vi "Main.vi"() -> ()   [LabVIEW 2010]
uses:
  <vilib>/Utility/miscctls.llb/LVMenuShortCut.ctl
  sub VIs v Hauptprogramm/globale Variable 1.vi
panel:
  out "version":string="1.5.1.1"
  in  "Stopp 2":bool
  in  "endgültigeschließung":bool
  in  "fehlbearbeitungen":i32
  out "Farbwerte":T1
  in  "farbe":bool
  out "stop2":bool
  out "hitze":u64(knob)=398 caption="lichtquellen Temparatur" scale=420.0..356.0
  in  "Not-Aus betätigt":dbl
  in  "bearbeitung gestartedt":dbl
  out "start zeit":timestamp
  in  "protokoll":bool
  out "Lampe Notaus":bool
  out "error out":errorcluster
  in  "pneutest":bool
  out "error out senke":errorcluster
  out "gesperrt?":bool
  in  "schließen":bool
  out "export?":bool
  in  "error in (no error)":errorcluster caption="Fehler (Eingang, kein Fehler)"
  in  "Licht":bool
  in  "Ende":bool
  out "Device ID Out":T2(ring)
  in  "Interfacetest":bool
  in  "Stopp":bool
  out "Zeitstempel":timestamp=timestamp(-9593251200 s since 1904-01-01) format="%<%H:%M:%S\n%d/%m/%Y>T"
  in  "Sperren":bool
  # "456"
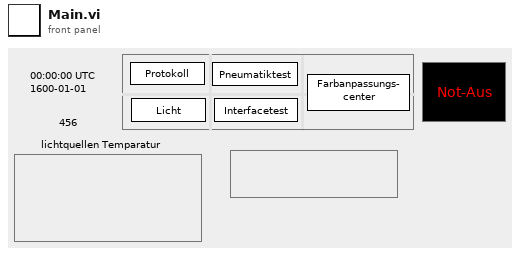
[diagram p1: front panel]
types:
  T1 = cluster{"Rot-min.":dbl, "Rot.max.":dbl, "Blau-min.":dbl, "Blau-max.":dbl, "Grün-min.":dbl, "Grün-max.":dbl, "Weiß-min.":dbl, "Weiß-max.":dbl}
  T2 = enum16{"Device 1", "Device 2", "Device 3", "Device 4", "Device 5", "Device 6", "Device 7", "Device 8"}
  T3 = enum8{"Power 1", "Power 2", "Power 3", "Power 4", "Power 5", "Power 6", "Power 7", "Power 8"}
  T4 = enum8{"Output 1 (O1)", "Output 2 (O2)", "Output 3 (O3)", "Output 4 (O4)", "Output 5 (O5)", "Output 6 (O6)", "Output 7 (O7)", "Output 8 (O8)"}
  T5 = enum8{"Robo Interface", "Extension 1", "Extension 2", "Extension 3"}
  T6 = enum8{"Input 1 (I1)", "Input 2 (I2)", "Input 3 (I3)", "Input 4 (I4)", "Input 5 (I5)", "Input 6 (I6)", "Input 7 (I7)", "Input 8 (I8)"}
  T7 = enum8{"Input AX", "Input AY", "Input A1", "Input A2", "Input AZ", "Input AV", "Input D1", "Input D2", "Input AXR", "Input AYR"}
  T8 = enum8{"Goes High", "Goes Low", "Goes High or Low"}
  T9 = typedef "LVMenuShortCut.ctl" = cluster{"Include Shift Key?":bool, "Include Ctrl Key?":bool, "Shortcut Key":string}
  T10 = enum8{"Robo Interface", "Extension 1", "Extension 2", "Extension 3"}[]
  T11 = enum8{"Input 1 (I1)", "Input 2 (I2)", "Input 3 (I3)", "Input 4 (I4)", "Input 5 (I5)", "Input 6 (I6)", "Input 7 (I7)", "Input 8 (I8)"}[]
  T12 = cluster{"Value[0]":bool, "Value[1]":bool, "Value[2]":bool, "Value[3]":bool, "Value[4]":bool, "Value[5]":bool, "Value[6]":bool, "Value[7]":bool, "Value[8]":bool}
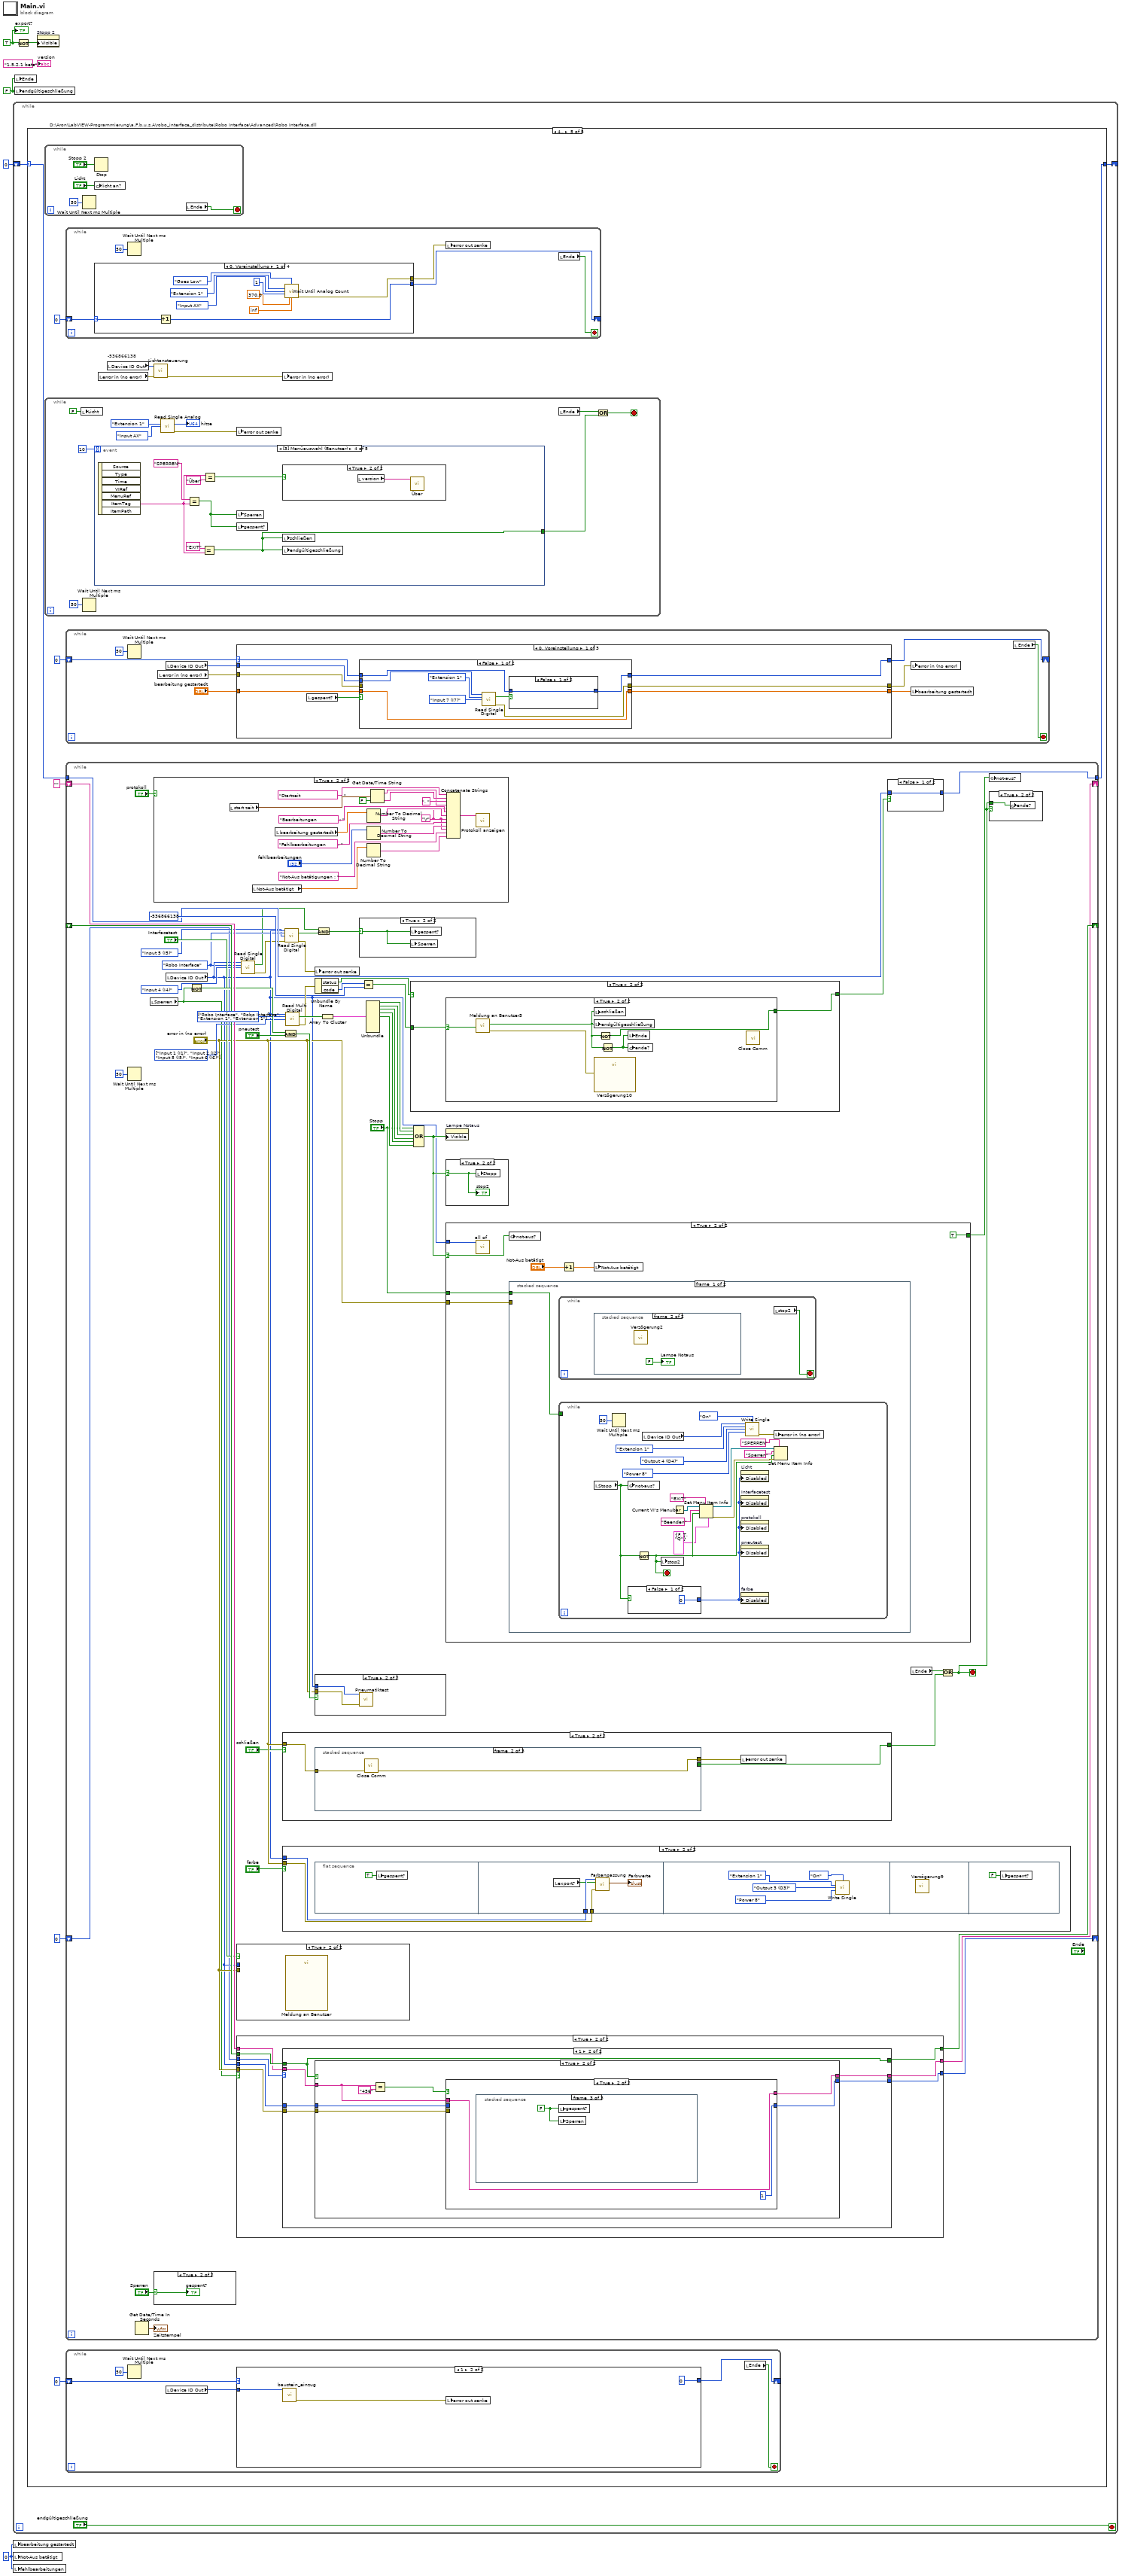
[diagram p0: block diagram]
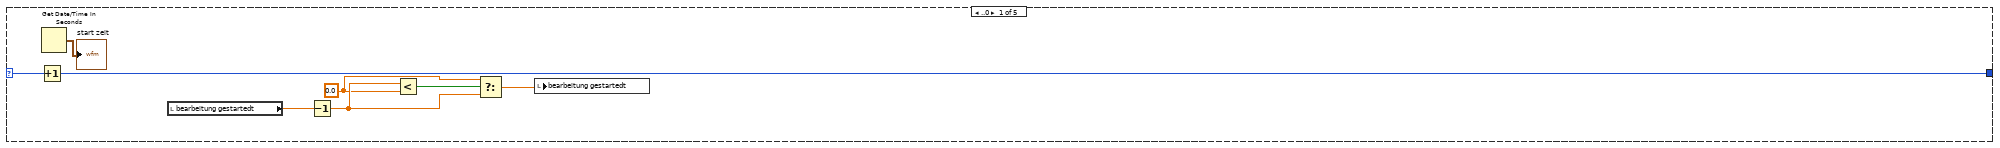
[diagram p2: hidden frame]
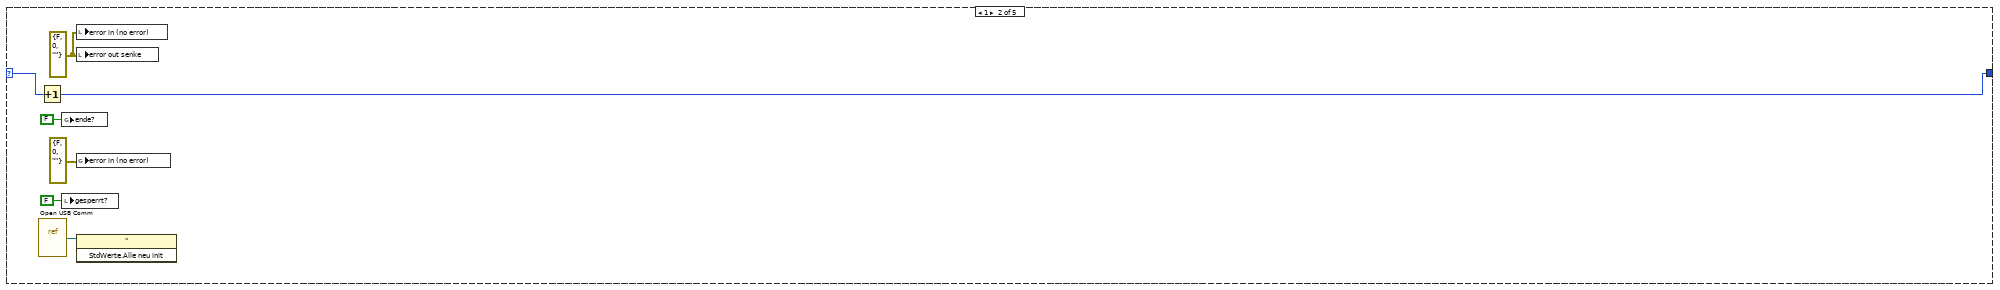
[diagram p3: hidden frame]
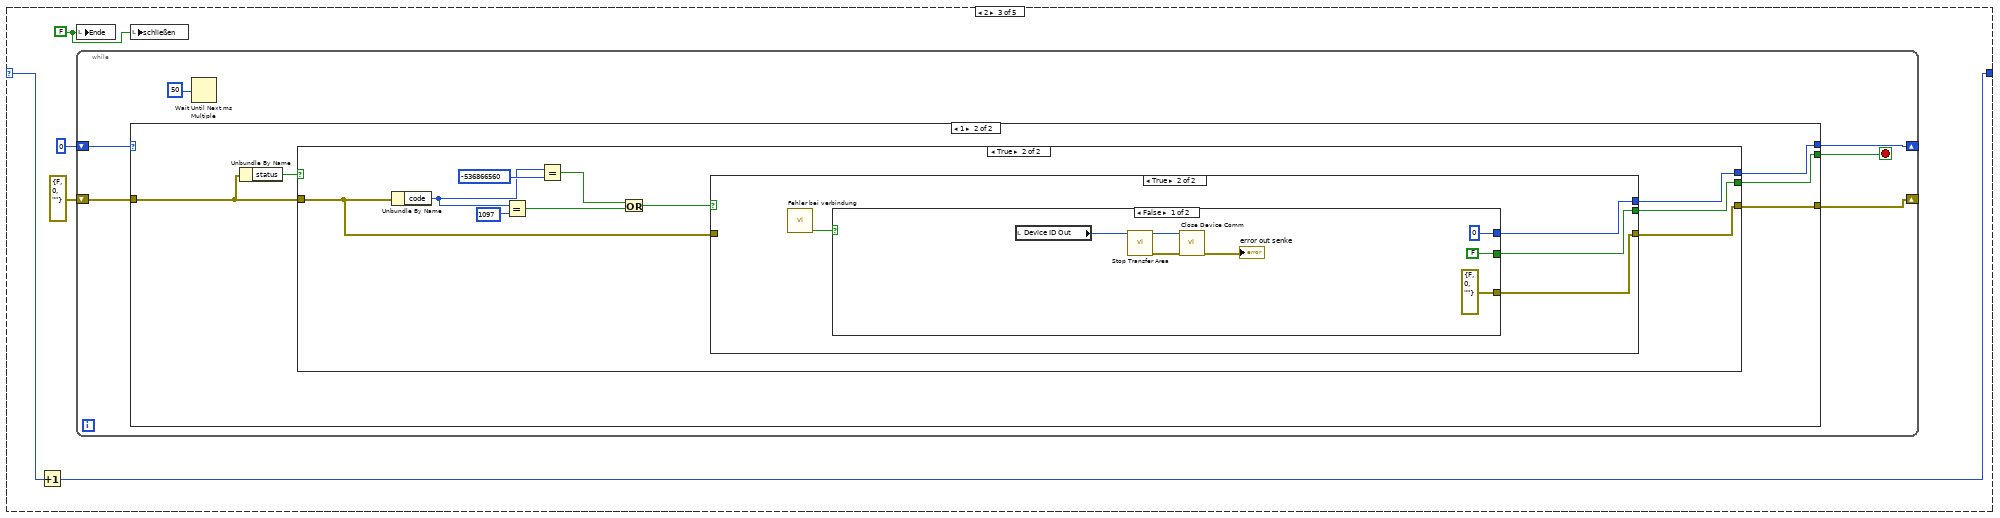
[diagram p4: hidden frame]
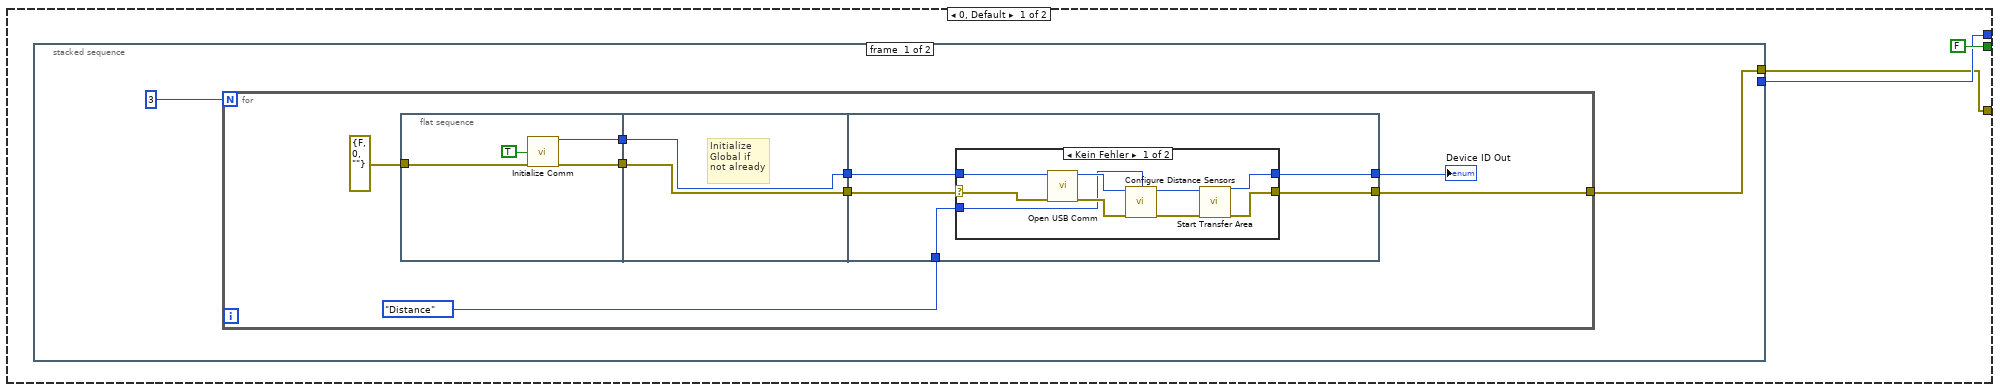
[diagram p5: hidden frame]
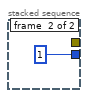
[diagram p7: hidden frame]
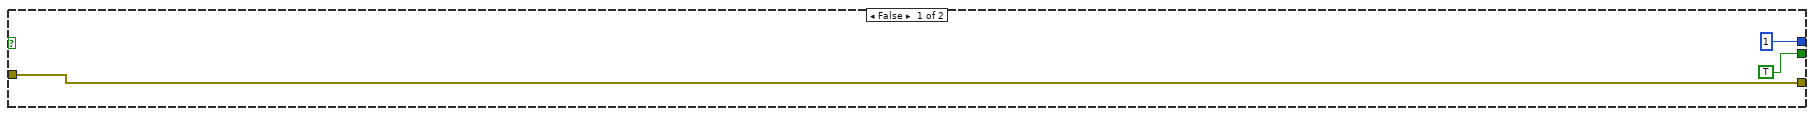
[diagram p8: hidden frame]
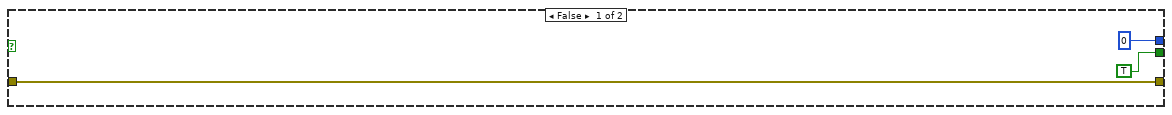
[diagram p9: hidden frame]
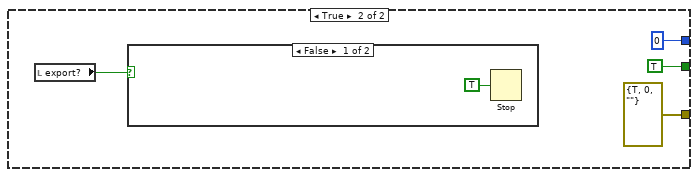
[diagram p10: hidden frame]
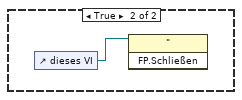
[diagram p11: hidden frame]
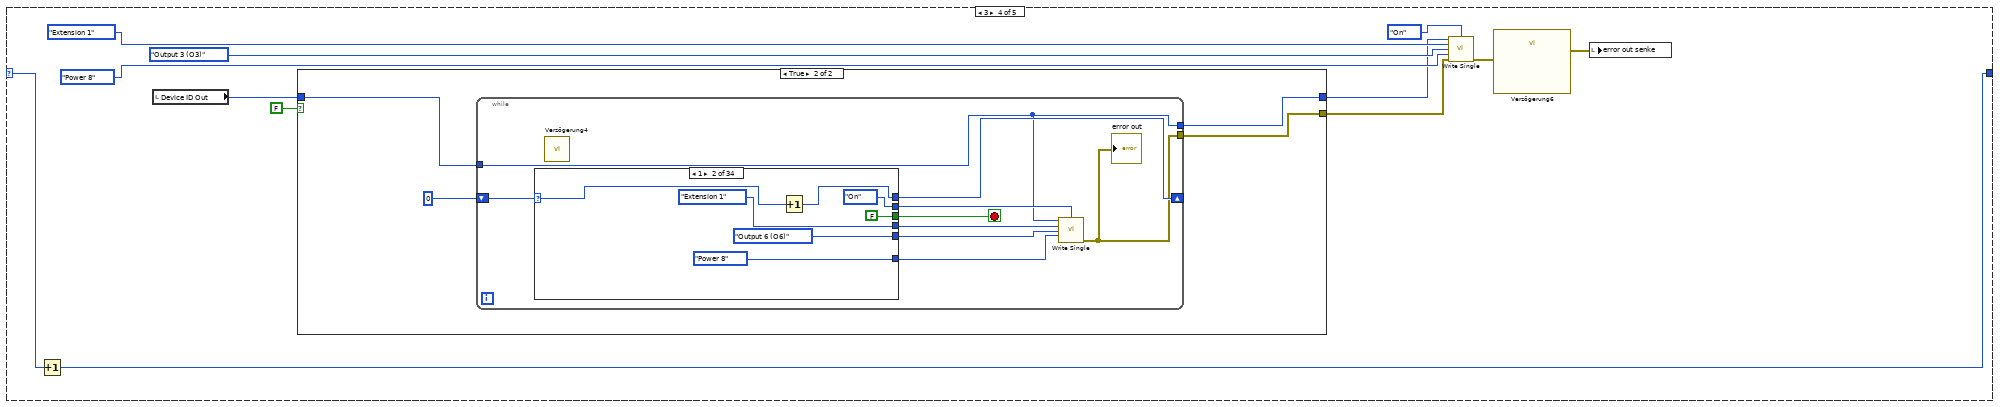
[diagram p12: hidden frame]
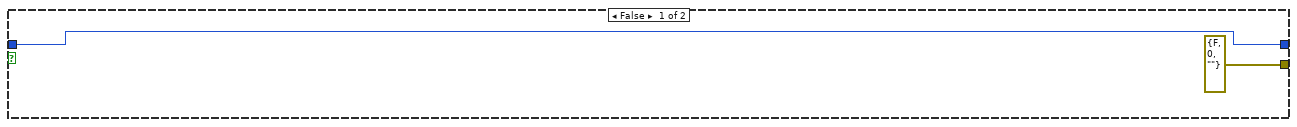
[diagram p13: hidden frame]
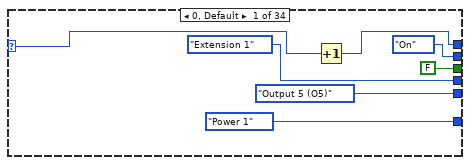
[diagram p14: hidden frame]
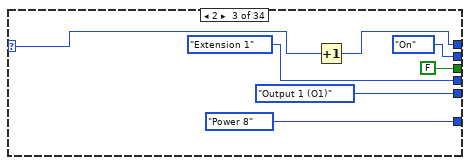
[diagram p15: hidden frame]
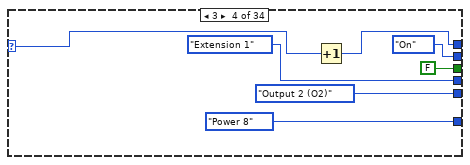
[diagram p16: hidden frame]
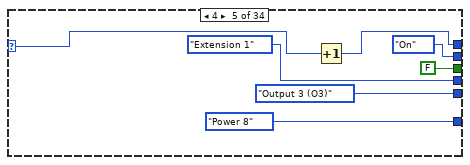
[diagram p17: hidden frame]
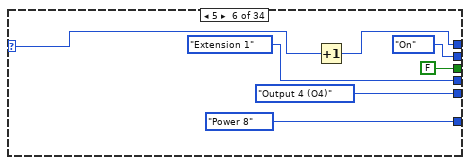
[diagram p18: hidden frame]
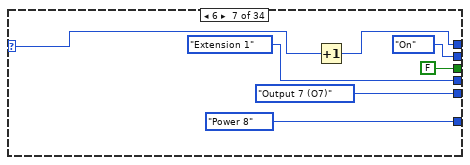
[diagram p19: hidden frame]
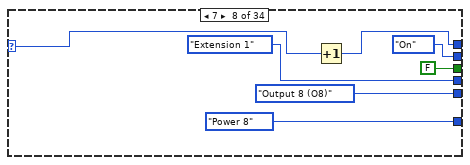
[diagram p20: hidden frame]
diagram:
  w4 = 0
  w5 = FALSE ("Ende")
  w3 = TRUE ("export?")
  n1 = while {
    shift-right: [w7] -> _
    shift-left: 0 -> [w9]
    stop <- "endgültigeschließung" stop-if-true
    # "D:\\Aron\\LabVIEW-Programmierung\\a.F.b.u.s.A\\robo_interface_distribute\\Robo Interface\\Advanced\\Robo Interface.dll"
    n2 = case shown="4.." w9 {
      selector: w9 -> [w16 w20 w25 w112 w376]
      tunnel: [w15 w19 w26 w111 w375] -> w7
      frame ..0 {
        w11 = 0.0 ("y")
        n3 = Increment(x=w16) -> (x+1=w15:i32)
        n4 = Get Date/Time In Seconds() -> (seconds since 1Jan1904=→"start zeit":timestamp)
        n5 = local read "bearbeitung gestartedt"() -> (w14:dbl)
        n6 = Decrement(x=w14) -> (x-1=w12:dbl)
        n7 = Less?(x=w12, y=w11) -> (x < y?=w13:bool)
        n8 = Select(t=w11, s=w13, f=w12) -> (s? t:f=w10:dbl)
        n9 = local write "bearbeitung gestartedt"(w10) -> ()
      }
      frame 1 {
        w21 = errorcluster {"status"=FALSE, "code"=0, "source"=""} ("error in (no error)")
        n10 = vi-ref "Open USB Comm.vi"() -> (w24:refnum<vi>)
        n11 = Increment(x=w20) -> (x+1=w19:i32)
        n12 = global write "globale Variable 1.vi" "ende?"(FALSE ("ende?")) -> ()
        n13 = local write "gesperrt?"(FALSE ("gesperrt?")) -> ()
        n14 = local write "error in (no error)"(w21) -> ()
        n15 = local write "error out senke"(w21) -> ()
        n16 = global write "globale Variable 1.vi" "error in (no error)"(errorcluster {"status"=FALSE, "code"=0, "source"=""} ("error in (no error)")) -> ()
        n17 = invoke class="\"" method="StdWerte.Alle neu init"(reference=w24) -> ()  [unwired: 2 in, 3 out]
      }
      frame 2 {
        w27 = FALSE
        n18 = Increment(x=w25) -> (x+1=w26:i32)
        n19 = local write "Ende"(w27) -> ()
        n20 = while {
          shift-right: [w32] -> _
          shift-left: 0 -> [w35]
          shift-right: [w34] -> _
          shift-left: errorcluster {"status"=FALSE, "code"=0, "source"=""} ("error out") -> [w33]
          stop <- w31 stop-if-true
          n21 = case shown="1" w35 {
            tunnel: [w36 w72] -> w34
            tunnel: w33 -> [_ w73]
            tunnel: [w37 w76] -> w32
            tunnel: [FALSE w74] -> w31
            frame 0, Default {
              n22 = stacked-sequence {
                tunnel: [_ 1] -> w37
                tunnel: [w40 _] -> w36
                frame #0 {
                  n23 = for {
                    N: 3 -> [_]
                    tunnel: [w41] -> w40
                    n24 = flat-sequence {
                      tunnel: [w52] -> w48
                      tunnel: [w51] -> w47
                      tunnel: errorcluster {"status"=FALSE, "code"=0, "source"=""} ("error in") -> [w50]
                      tunnel: [w54] -> w46
                      tunnel: [w53] -> w45
                      tunnel: w48 -> [w54]
                      tunnel: w47 -> [w53]
                      tunnel: w46 -> [w59]
                      tunnel: w45 -> [w58]
                      tunnel: [w57] -> w41
                      tunnel: [w56] -> w44
                      tunnel: enum32{"Voltage", "Distance"}."Distance" ("Distance Sensor Mode") -> [w55]
                      frame #0 {
                        n25 = call "Initialize Comm.vi"("immer erster aufruf?"=TRUE, "error in"=w50) -> ("Device ID Out"=w52:T2, "error out"=w51:errorcluster)  [unwired: 1 in, 11 out]
                      }
                      frame #1 {
                        # "Initialize\nGlobal if\nnot already"
                      }
                      frame #2 {
                        n26 = case shown="Kein Fehler" w58 {
                          selector: w58 -> [w65 w70]
                          tunnel: [w68 w70] -> w57
                          tunnel: w59 -> [w63 w69]
                          tunnel: [w67 w69] -> w56
                          tunnel: w55 -> [w61 _]
                          frame No Error {
                            n27 = call "Open USB Comm.vi"("Device ID"=w63, "error in"=w65) -> ("Device ID Out"=w62:T2, "error out"=w64:errorcluster)  [unwired: 12 out]
                            n28 = call "Configure Distance Sensors.vi"("Device ID"=w62, "Distance Sensor Mode"=w61, "error in"=w64) -> ("Device ID Out"=w60:T2, "error out"=w66:errorcluster)  [unwired: 6 in, 5 out]
                            n29 = call "Start Transfer Area.vi"("Device ID"=w60, "error in"=w66) -> ("Device ID Out"=w67:T2, "error out"=w68:errorcluster)  [unwired: 12 out]
                          }
                          frame Error {
                          }
                        }
                      }
                    }
                    "Device ID Out" <- w44
                  }
                }
                frame #1 {
                }
              }
            }
            frame 1 {
              n30 = Unbundle By Name(w73) -> ("status"=w75:bool)
              n31 = case shown="True" w75 {
                tunnel: w73 -> [w77 w88]
                tunnel: [1 w87] -> w76
                tunnel: [TRUE w86] -> w74
                tunnel: [w77 w85] -> w72
                frame False {
                }
                frame True {
                  n32 = Unbundle By Name(w88) -> ("code"=w84:i32)
                  n33 = Equal?(x=w84, y=1097) -> (x = y?=w82:bool)
                  n34 = Equal?(x=w84, y=-536866560) -> (x = y?=w83:bool)
                  n35 = Or(x=w83, y=w82) -> (x .or. y?=w81:bool)
                  n36 = case shown="True" w81 {
                    tunnel: w88 -> [w90 _]
                    tunnel: [0 w96] -> w87
                    tunnel: [TRUE w95] -> w86
                    tunnel: [w90 w94] -> w85
                    frame False {
                    }
                    frame True {
                      n37 = call "Fehler bei verbindung.vi"() -> ("schließen?"=w93:bool)  [unwired: 11 out]
                      n38 = case shown="False" w93 {
                        tunnel: [0 0] -> w96
                        tunnel: [FALSE TRUE] -> w95
                        tunnel: [errorcluster {"status"=FALSE, "code"=0, "source"=""} ("error out") errorcluster {"status"=TRUE, "code"=0, "source"=""} ("error out")] -> w94
                        frame False {
                          n39 = local read "Device ID Out"() -> (w99:T2)
                          n40 = call "Stop Transfer Area.vi"("Device ID"=w99) -> ("Device ID Out"=w100:T2, "error out"=w97:errorcluster)  [unwired: 1 in, 12 out]
                          n41 = call "Close Device Comm.vi"("Device ID"=w100, "error in"=w97) -> ("error out"=→"error out senke":errorcluster)  [unwired: 13 out]
                        }
                        frame True {
                          n42 = local read "export?"() -> (w104:bool)
                          n43 = case shown="False" w104 {
                            frame False {
                              n44 = Stop(stop? (T)=TRUE ("Stopp? (T)")) -> ()
                            }
                            frame True {
                              n45 = control-ref of="dieses VI"() -> (w109:refnum<vi>)
                              n46 = invoke class="\"" method="FP.Schließen"(reference=w109) -> ()  [unwired: 2 in, 3 out]
                            }
                          }
                        }
                      }
                    }
                  }
                }
              }
            }
          }
          n47 = Wait Until Next ms Multiple(millisecond multiple=50) -> ()  [unwired: 1 out]
        }
        n48 = local write "schließen"(w27) -> ()
      }
      frame 3 {
        n49 = Increment(x=w112) -> (x+1=w111:i32)
        n50 = local read "Device ID Out"() -> (w115:T2)
        n51 = case shown="True" FALSE {
          tunnel: [w123 w126] -> w118
          tunnel: [errorcluster {"status"=FALSE, "code"=0, "source"=""} ("error out") w125] -> w117
          tunnel: w115 -> [w123 w124]
          frame False {
          }
          frame True {
            n52 = while {
              shift-right: [w131] -> _
              shift-left: 0 -> [w136]
              tunnel: [w128] -> w126
              tunnel: [w129] -> w125
              tunnel: w124 -> [w128]
              stop <- w130 stop-if-true
              n53 = case shown="1" w136 {
                selector: w136 -> [w139 w146 w153 w160 w167 w174 w181 w188 w195 w202 w209 w216 w223 w230 w237 w244 w251 w258 w265 w272 w279 w286 w293 w300 w307 w314 w321 w328 w335 w342 w349 w356 w363 w370]
                tunnel: [T3."Power 1" ("Output_PWM") T3."Power 8" ("Output_PWM") T3."Power 8" ("Output_PWM") T3."Power 8" ("Output_PWM") T3."Power 8" ("Output_PWM") T3."Power 8" ("Output_PWM") T3."Power 8" ("Output_PWM") T3."Power 8" ("Output_PWM") T3."Power 1" ("Output_PWM") T3."Power 8" ("Output_PWM") T3."Power 8" ("Output_PWM") T3."Power 8" ("Output_PWM") T3."Power 8" ("Output_PWM") T3."Power 8" ("Output_PWM") T3."Power 1" ("Output_PWM") T3."Power 4" ("Output_PWM") T3."Power 8" ("Output_PWM") T3."Power 8" ("Output_PWM") T3."Power 8" ("Output_PWM") T3."Power 8" ("Output_PWM") T3."Power 8" ("Output_PWM") T3."Power 8" ("Output_PWM") T3."Power 8" ("Output_PWM") T3."Power 4" ("Output_PWM") T3."Power 8" ("Output_PWM") T3."Power 8" ("Output_PWM") T3."Power 8" ("Output_PWM") T3."Power 8" ("Output_PWM") T3."Power 8" ("Output_PWM") T3."Power 8" ("Output_PWM") T3."Power 8" ("Output_PWM") T3."Power 8" ("Output_PWM") T3."Power 8" ("Output_PWM") T3."Power 1" ("Output_PWM")] -> w135
                tunnel: [T4."Output 5 (O5)" ("Single_Output") T4."Output 6 (O6)" ("Single_Output") T4."Output 1 (O1)" ("Single_Output") T4."Output 2 (O2)" ("Single_Output") T4."Output 3 (O3)" ("Single_Output") T4."Output 4 (O4)" ("Single_Output") T4."Output 7 (O7)" ("Single_Output") T4."Output 8 (O8)" ("Single_Output") T4."Output 5 (O5)" ("Single_Output") T4."Output 6 (O6)" ("Single_Output") T4."Output 1 (O1)" ("Single_Output") T4."Output 2 (O2)" ("Single_Output") T4."Output 3 (O3)" ("Single_Output") T4."Output 4 (O4)" ("Single_Output") T4."Output 5 (O5)" ("Single_Output") T4."Output 7 (O7)" ("Single_Output") T4."Output 8 (O8)" ("Single_Output") T4."Output 1 (O1)" ("Single_Output") T4."Output 2 (O2)" ("Single_Output") T4."Output 3 (O3)" ("Single_Output") T4."Output 4 (O4)" ("Single_Output") T4."Output 5 (O5)" ("Single_Output") T4."Output 6 (O6)" ("Single_Output") T4."Output 7 (O7)" ("Single_Output") T4."Output 8 (O8)" ("Single_Output") T4."Output 1 (O1)" ("Single_Output") T4."Output 2 (O2)" ("Single_Output") T4."Output 3 (O3)" ("Single_Output") T4."Output 4 (O4)" ("Single_Output") T4."Output 5 (O5)" ("Single_Output") T4."Output 6 (O6)" ("Single_Output") T4."Output 7 (O7)" ("Single_Output") T4."Output 8 (O8)" ("Single_Output") T4."Output 5 (O5)" ("Single_Output")] -> w134
                tunnel: [T5."Extension 1" ("Module") T5."Extension 1" ("Module") T5."Extension 1" ("Module") T5."Extension 1" ("Module") T5."Extension 1" ("Module") T5."Extension 1" ("Module") T5."Extension 1" ("Module") T5."Extension 1" ("Module") T5."Extension 1" ("Module") T5."Extension 1" ("Module") T5."Extension 1" ("Module") T5."Extension 1" ("Module") T5."Extension 1" ("Module") T5."Extension 1" ("Module") T5."Extension 1" ("Module") T5."Extension 1" ("Module") T5."Extension 1" ("Module") T5."Robo Interface" ("Module") T5."Robo Interface" ("Module") T5."Robo Interface" ("Module") T5."Robo Interface" ("Module") T5."Robo Interface" ("Module") T5."Robo Interface" ("Module") T5."Robo Interface" ("Module") T5."Robo Interface" ("Module") T5."Robo Interface" ("Module") T5."Robo Interface" ("Module") T5."Robo Interface" ("Module") T5."Robo Interface" ("Module") T5."Robo Interface" ("Module") T5."Robo Interface" ("Module") T5."Robo Interface" ("Module") T5."Robo Interface" ("Module") T5."Extension 1" ("Module")] -> w133
                tunnel: [enum8{"Off", "On"}."On" ("Output_Action") enum8{"Off", "On"}."On" ("Output_Action") enum8{"Off", "On"}."On" ("Output_Action") enum8{"Off", "On"}."On" ("Output_Action") enum8{"Off", "On"}."On" ("Output_Action") enum8{"Off", "On"}."On" ("Output_Action") enum8{"Off", "On"}."On" ("Output_Action") enum8{"Off", "On"}."On" ("Output_Action") enum8{"Off", "On"}."Off" ("Output_Action") enum8{"Off", "On"}."Off" ("Output_Action") enum8{"Off", "On"}."Off" ("Output_Action") enum8{"Off", "On"}."Off" ("Output_Action") enum8{"Off", "On"}."Off" ("Output_Action") enum8{"Off", "On"}."Off" ("Output_Action") enum8{"Off", "On"}."Off" ("Output_Action") enum8{"Off", "On"}."Off" ("Output_Action") enum8{"Off", "On"}."Off" ("Output_Action") enum8{"Off", "On"}."On" ("Output_Action") enum8{"Off", "On"}."On" ("Output_Action") enum8{"Off", "On"}."On" ("Output_Action") enum8{"Off", "On"}."On" ("Output_Action") enum8{"Off", "On"}."On" ("Output_Action") enum8{"Off", "On"}."On" ("Output_Action") enum8{"Off", "On"}."On" ("Output_Action") enum8{"Off", "On"}."On" ("Output_Action") enum8{"Off", "On"}."Off" ("Output_Action") enum8{"Off", "On"}."Off" ("Output_Action") enum8{"Off", "On"}."Off" ("Output_Action") enum8{"Off", "On"}."Off" ("Output_Action") enum8{"Off", "On"}."Off" ("Output_Action") enum8{"Off", "On"}."Off" ("Output_Action") enum8{"Off", "On"}."Off" ("Output_Action") enum8{"Off", "On"}."Off" ("Output_Action") enum8{"Off", "On"}."Off" ("Output_Action")] -> w132
                tunnel: [w138 w145 w152 w159 w166 w173 w180 w187 w194 w201 w208 w215 w222 w229 w236 w243 w250 w257 w264 w271 w278 w285 w292 w299 w306 w313 w320 w327 w334 w341 w348 w355 w362 w369] -> w131
                tunnel: [FALSE FALSE FALSE FALSE FALSE FALSE FALSE FALSE FALSE FALSE FALSE FALSE FALSE FALSE FALSE FALSE FALSE FALSE FALSE FALSE FALSE FALSE FALSE FALSE FALSE FALSE FALSE FALSE FALSE FALSE FALSE FALSE FALSE TRUE] -> w130
                frame 0, Default {
                  n54 = Increment(x=w139) -> (x+1=w138:i32)
                }
                frame 1 {
                  n55 = Increment(x=w146) -> (x+1=w145:i32)
                }
                frame 2 {
                  n56 = Increment(x=w153) -> (x+1=w152:i32)
                }
                frame 3 {
                  n57 = Increment(x=w160) -> (x+1=w159:i32)
                }
                frame 4 {
                  n58 = Increment(x=w167) -> (x+1=w166:i32)
                }
                frame 5 {
                  n59 = Increment(x=w174) -> (x+1=w173:i32)
                }
                frame 6 {
                  n60 = Increment(x=w181) -> (x+1=w180:i32)
                }
                frame 7 {
                  n61 = Increment(x=w188) -> (x+1=w187:i32)
                }
                frame 8 {
                  n62 = Increment(x=w195) -> (x+1=w194:i32)
                }
                frame 9 {
                  n63 = Increment(x=w202) -> (x+1=w201:i32)
                }
                frame 10 {
                  n64 = Increment(x=w209) -> (x+1=w208:i32)
                }
                frame 11 {
                  n65 = Increment(x=w216) -> (x+1=w215:i32)
                }
                frame 12 {
                  n66 = Increment(x=w223) -> (x+1=w222:i32)
                }
                frame 13 {
                  n67 = Increment(x=w230) -> (x+1=w229:i32)
                }
                frame 14 {
                  n68 = Increment(x=w237) -> (x+1=w236:i32)
                }
                frame 15 {
                  n69 = Increment(x=w244) -> (x+1=w243:i32)
                }
                frame 16 {
                  n70 = Increment(x=w251) -> (x+1=w250:i32)
                }
                frame 17 {
                  n71 = Increment(x=w258) -> (x+1=w257:i32)
                }
                frame 18 {
                  n72 = Increment(x=w265) -> (x+1=w264:i32)
                }
                frame 19 {
                  n73 = Increment(x=w272) -> (x+1=w271:i32)
                }
                frame 20 {
                  n74 = Increment(x=w279) -> (x+1=w278:i32)
                }
                frame 21 {
                  n75 = Increment(x=w286) -> (x+1=w285:i32)
                }
                frame 22 {
                  n76 = Increment(x=w293) -> (x+1=w292:i32)
                }
                frame 23 {
                  n77 = Increment(x=w300) -> (x+1=w299:i32)
                }
                frame 24 {
                  n78 = Increment(x=w307) -> (x+1=w306:i32)
                }
                frame 25 {
                  n79 = Increment(x=w314) -> (x+1=w313:i32)
                }
                frame 26 {
                  n80 = Increment(x=w321) -> (x+1=w320:i32)
                }
                frame 27 {
                  n81 = Increment(x=w328) -> (x+1=w327:i32)
                }
                frame 29 {
                  n82 = Increment(x=w335) -> (x+1=w334:i32)
                }
                frame 30 {
                  n83 = Increment(x=w342) -> (x+1=w341:i32)
                }
                frame 31 {
                  n84 = Increment(x=w349) -> (x+1=w348:i32)
                }
                frame 32 {
                  n85 = Increment(x=w356) -> (x+1=w355:i32)
                }
                frame 33 {
                  n86 = Increment(x=w363) -> (x+1=w362:i32)
                }
                frame 34 {
                  n87 = Increment(x=w370) -> (x+1=w369:i32)
                }
              }
              n88 = call "Verzögerung4"() -> ()  [unwired: 2 in, 10 out]
              n89 = call "Write Single.vi"("Device ID"=w128, "Output_Action"=w132, "Module"=w133, "Single_Output"=w134, "Output_PWM"=w135) -> ("error out"=w129:errorcluster)  [unwired: 1 in, 9 out]
              "error out" <- w129
            }
          }
        }
        n90 = call "Write Single.vi"("Device ID"=w118, "Output_Action"=enum8{"Off", "On"}."On", "Module"=T5."Extension 1", "Single_Output"=T4."Output 3 (O3)", "Output_PWM"=T3."Power 8", "error in"=w117) -> ("error out"=w113:errorcluster)  [unwired: 9 out]
        n91 = call "Verzögerung6"("error in (no error)"=w113) -> ("error out"=w110:errorcluster)  [unwired: 1 in, 9 out]
        n92 = local write "error out senke"(w110) -> ()
      }
      frame 4.. {
        # "-536866138"
        n93 = while {
          stop <- w436 stop-if-true
          n94 = Wait Until Next ms Multiple(millisecond multiple=50) -> ()  [unwired: 1 out]
          n95 = Stop(stop? (T)="Stopp 2") -> ()
          n96 = global write "globale Variable 1.vi" "licht an?"("Licht") -> ()
          n97 = local read "Ende"() -> (w436:bool)
        }
        n98 = while {
          stop <- w413 stop-if-true
          n99 = local write "Licht"(FALSE) -> ()
          n100 = Wait Until Next ms Multiple(millisecond multiple=50) -> ()  [unwired: 1 out]
          n101 = event shown="[3] Menüauswahl (Benutzer)" {
            selector: _ -> [_ _ _ _ _]
            dyn-events: _ -> [_ _ _ _ _]
            timeout: 10 -> [_ _ _ _ _]
            tunnel: [TRUE w421 FALSE ("Ende") w427 w432] -> w414
            event Panel Close? {
              w418 = TRUE ("schließen")
              n102 = event-data() -> ()  [unwired: 4 out]
              n103 = local write "schließen"(w418) -> ()
              n104 = local write "endgültigeschließung"(w418) -> ()
              n105 = event-data("Discard?"=TRUE ("Verwerfen?")) -> ()  [unwired: 1 in, 1 out]
            }
            event "Ende": Value Change {
              n106 = event-data() -> ("NewVal"=w421:bool)  [unwired: 6 out]
            }
            event Shortcut Menu Activation? {
              n107 = event-data() -> ("MenuRef"=w423:refnum<k9>)  [unwired: 7 out]
              n108 = Delete Menu Items(9:w423) -> ()  [unwired: 1 in, 4 out]
              n109 = event-data() -> ()  [unwired: 1 in, 2 out]
            }
            event Menu Selection (User) {
              n110 = event-data() -> ("ItemTag"=w426:string)  [unwired: 7 out]
              n111 = Equal?(x="SPERREN", y=w426) -> (x = y?=w428:bool)
              n112 = Equal?(x="EXIT", y=w426) -> (x = y?=w427:bool)
              n113 = Equal?(x=w426, y="Über") -> (x = y?=w424:bool)
              n114 = local write "Sperren"(w428) -> ()
              n115 = local write "gesperrt?"(w428) -> ()
              n116 = case shown="True" w424 {
                frame False {
                }
                frame True {
                  n117 = local read "version"() -> (w431:string)
                  n118 = call "Über.vi"("version"=w431) -> ()  [unwired: 11 out]
                }
              }
              n119 = local write "schließen"(w427) -> ()
              n120 = local write "endgültigeschließung"(w427) -> ()
            }
            event Timeout {
              n121 = event-data() -> ()  [unwired: 4 out]
              n122 = local read "Ende"() -> (w432:bool)
            }
          }
          n123 = call "Read Single Analog.vi"("Module"=T5."Extension 1", "Analog_Input"=T7."Input AX") -> ("Value"=→"hitze":u16, "error out"=w408:errorcluster)  [unwired: 2 in, 10 out]
          n124 = local write "error out senke"(w408) -> ()
          n125 = local read "Ende"() -> (w416:bool)
          n126 = Or(x=w416, y=w414) -> (x .or. y?=w413:bool)
        }
        n127 = while {
          shift-right: [w502] -> _
          shift-left: 0 -> [w503]
          stop <- w504 stop-if-true
          n128 = case shown="0, Voreinstellung" w503 {
            selector: w503 -> [w508 w516 w529 _]
            tunnel: [w507 w517 w530 0] -> w502
            tunnel: [w509 w515 w523 w531] -> w501
            frame 0, Default {
              n129 = Increment(x=w508) -> (x+1=w507:i32)
              n130 = call "Wait Until Analog Count.vi"("Wait Until"=T8."Goes Low", "Module"=T5."Extension 1", "Analog_Input"=T7."Input AX", "Final Count"=u32 1, "Level"=370.0, "Time Out (10)"=inf) -> ("error out"=w509:errorcluster)  [unwired: 2 in, 7 out]
            }
            frame 1 {
              n131 = Increment(x=w516) -> (x+1=w517:i32)
              n132 = call "Write Single.vi"("Output_Action"=enum8{"Off", "On"}."On", "Module"=T5."Robo Interface", "Single_Output"=T4."Output 4 (O4)", "Output_PWM"=T3."Power 8") -> ("error out"=w515:errorcluster)  [unwired: 2 in, 9 out]
            }
            frame 2 {
              n133 = Increment(x=w529) -> (x+1=w530:i32)
              n134 = call "Wait Until Analog Count.vi"("Wait Until"=T8."Goes High", "Module"=T5."Extension 1", "Analog_Input"=T7."Input AX", "Final Count"=u32 1, "Level"=415.0, "Time Out (10)"=inf) -> ("error out"=w523:errorcluster)  [unwired: 2 in, 7 out]
            }
            frame 3 {
              n135 = call "Write Single.vi"("Output_Action"=enum8{"Off", "On"}."Off", "Module"=T5."Robo Interface", "Single_Output"=T4."Output 4 (O4)") -> ("error out"=w531:errorcluster)  [unwired: 3 in, 9 out]
            }
          }
          n136 = Wait Until Next ms Multiple(millisecond multiple=50) -> ()  [unwired: 1 out]
          n137 = local write "error out senke"(w501) -> ()
          n138 = local read "Ende"() -> (w504:bool)
        }
        n139 = while {
          shift-right: [w439] -> _
          shift-left: 0 -> [w440]
          stop <- w445 stop-if-true
          n140 = Wait Until Next ms Multiple(millisecond multiple=50) -> ()  [unwired: 1 out]
          n141 = local read "error in (no error)"() -> (w442:errorcluster)
          n142 = local read "Device ID Out"() -> (w443:T2)
          n143 = case shown="0, Voreinstellung" w440 {
            selector: w440 -> [w446 w475 _]
            tunnel: w443 -> [w451 w472 w496]
            tunnel: w442 -> [w450 w471 w490]
            tunnel: [w452 w473 w498] -> w441
            tunnel: [w453 w474 0] -> w439
            tunnel: [w448 w469 w494] -> w437
            tunnel: "bearbeitung gestartedt" -> [w447 w468 w493]
            frame 0, Default {
              n144 = local read "gesperrt?"() -> (w449:bool)
              n145 = case shown="False" w449 {
                tunnel: w446 -> [w461 w467]
                tunnel: [w460 w467] -> w453
                tunnel: [w455 w466] -> w452
                tunnel: w451 -> [w456 _]
                tunnel: w450 -> [_ w466]
                tunnel: [w459 w465] -> w448
                tunnel: w447 -> [w459 w465]
                frame False {
                  n146 = call "Read Single Digital.vi"("Device ID"=w456, "Module"=T5."Extension 1", "Digital_Input"=T6."Input 7 (I7)") -> ("Value"=w454:bool, "error out"=w455:errorcluster)  [unwired: 1 in, 10 out]
                  n147 = case shown="False" w454 {
                    tunnel: w461 -> [w462 w464]
                    tunnel: [w462 w463] -> w460
                    frame False {
                    }
                    frame True {
                      n148 = Increment(x=w464) -> (x+1=w463:i32)
                    }
                  }
                }
                frame True {
                }
              }
            }
            frame 1 {
              n149 = local read "gesperrt?"() -> (w470:bool)
              n150 = case shown="False" w470 {
                tunnel: w475 -> [w483 w489]
                tunnel: [w482 w489] -> w474
                tunnel: [w477 w488] -> w473
                tunnel: w472 -> [w478 _]
                tunnel: w471 -> [_ w488]
                tunnel: [w481 w487] -> w469
                tunnel: w468 -> [w481 w487]
                frame False {
                  n151 = call "Read Single Digital.vi"("Device ID"=w478, "Module"=T5."Extension 1", "Digital_Input"=T6."Input 7 (I7)") -> ("Value"=w476:bool, "error out"=w477:errorcluster)  [unwired: 1 in, 10 out]
                  n152 = case shown="False" w476 {
                    tunnel: w483 -> [w485 w486]
                    tunnel: [w484 w486] -> w482
                    frame False {
                      n153 = Increment(x=w485) -> (x+1=w484:i32)
                    }
                    frame True {
                    }
                  }
                }
                frame True {
                }
              }
            }
            frame 2 {
              n154 = Increment(x=w493) -> (x+1=w494:dbl)
              n155 = local read "Farbwerte"() -> (w492:T1)
              n156 = call "a.F.b.u.s.A bearbeiten.vi"("error in (no error)"=w490, "Farbwerte"=w492, "Stop?"=FALSE, "Device ID"=w496) -> ("error out"=w498:errorcluster, "fehlbarbeitung?"=w491:bool)  [unwired: 6 out]
              n157 = case shown="True" w491 {
                frame False {
                }
                frame True {
                  n158 = local read "fehlbearbeitungen"() -> (w499:i32)
                  n159 = Increment(x=w499) -> (x+1=w500:i32)
                  n160 = local write "fehlbearbeitungen"(w500) -> ()
                }
              }
            }
          }
          n161 = local write "error in (no error)"(w441) -> ()
          n162 = local write "bearbeitung gestartedt"(w437) -> ()
          n163 = local read "Ende"() -> (w445:bool)
        }
        n164 = while {
          shift-right: [w583] -> _
          shift-left: 0 -> [w536]
          shift-right: [w582] -> _
          shift-left: _ -> [w581]
          shift-right: [w579] -> _
          shift-left: "" -> [w577]
          tunnel: w376 -> [w553]
          tunnel: [w552] -> w375
          stop <- w548 stop-if-true
          w544 = T5."Robo Interface" ("Module")
          w571 = T10 [enum."Robo Interface", enum."Robo Interface", enum."Extension 1", enum."Extension 1"] items=["Robo Interface", "Extension 1", "Extension 2", "Extension 3"] ("Module")
          w573 = T11 [enum."Input 1 (I1)", enum."Input 2 (I2)", enum."Input 5 (I5)", enum."Input 6 (I6)"] items=["Input 1 (I1)", "Input 2 (I2)", "Input 3 (I3)", "Input 4 (I4)", "Input 5 (I5)", "Input 6 (I6)", "Input 7 (I7)", "Input 8 (I8)"] ("Digital Input")
          n165 = Wait Until Next ms Multiple(millisecond multiple=50) -> ()  [unwired: 1 out]
          n166 = Get Date/Time In Seconds() -> (seconds since 1Jan1904=→"Zeitstempel":timestamp)
          n167 = local read "Sperren"() -> (w537:bool)
          n168 = case shown="True" "protokoll" {
            frame False {
            }
            frame True {
              w614 = "\r"
              n169 = local read "start zeit"() -> (w628:timestamp)
              n170 = local read "Not-Aus betätigt"() -> (w619:dbl)
              n171 = local read "bearbeitung gestartedt"() -> (w622:dbl)
              n172 = Number To Decimal String(number=w622) -> (decimal integer string=w620:string)  [unwired: 1 out]
              n173 = Number To Decimal String(number="fehlbearbeitungen") -> (decimal integer string=w615:string)  [unwired: 1 out]
              n174 = Number To Decimal String(number=w619) -> (decimal integer string=w612:string)  [unwired: 1 out]
              n175 = Get Date/Time String(seconds (now)=w628, want seconds? (F)=FALSE ("Angabe von Sekunden? (F)")) -> (date string=w621:string, time string=w624:string)  [unwired: 1 out]
              n176 = Concatenate Strings("Startzeit                           : " ("String"), w624, ", " ("String"), w621, w614, "Bearbeitungen               : " ("String"), w620, w614, "Fehlbearbeitungen        : " ("String"), w615, w614, "Not-Aus betätigungen : " ("String"), w612) -> (w618:string)
              n177 = call "Protokoll anzeigen.vi"("String"=w618) -> ()  [unwired: 11 out]
            }
          }
          n178 = case shown="True" "Sperren" {
            selector: "Sperren" -> [_ w631]
            frame False {
            }
            frame True {
              "gesperrt?" <- w631
            }
          }
          n179 = local read "Device ID Out"() -> (w545:T2)
          n180 = Not(x=w537) -> (.not. x?=w575:bool)
          n181 = case shown="True" "Interfacetest" {
            tunnel: w545 -> [_ _]
            tunnel: "error in (no error)" -> [_ _]
            frame False {
            }
            frame True {
              n182 = call "Meldung an Benutzer"() -> ()  [unwired: 3 in, 9 out]
            }
          }
          n183 = case shown="True" w537 {
            tunnel: w536 -> [_ w656]
            tunnel: [0 w655] -> w583
            tunnel: [FALSE w654] -> w582
            tunnel: w581 -> [_ w653]
            tunnel: ["" w652] -> w579
            tunnel: w577 -> [_ w651]
            tunnel: w545 -> [_ w650]
            tunnel: "error in (no error)" -> [_ w649]
            frame False {
            }
            frame True {
              n184 = case shown="1" w656 {
                selector: w656 -> [w667 _]
                tunnel: [w666 w676] -> w655
                tunnel: [w665 w675] -> w654
                tunnel: w653 -> [_ w675]
                tunnel: [w668 w673] -> w652
                tunnel: w651 -> [_ w674]
                tunnel: w650 -> [_ w672]
                tunnel: w649 -> [_ w671]
                frame 0, Default {
                  n185 = call "Write Single.vi"("Output_Action"=enum8{"Off", "On"}."On", "Module"=T5."Extension 1", "Single_Output"=T4."Output 7 (O7)", "Output_PWM"=T3."Power 8") -> ()  [unwired: 2 in, 10 out]
                  n186 = call "Write Single.vi"("Output_Action"=enum8{"Off", "On"}."Off", "Module"=T5."Extension 1", "Single_Output"=T4."Output 3 (O3)", "Output_PWM"=T3."Power 8") -> ()  [unwired: 2 in, 10 out]
                  n187 = call "Passworteingabe.vi"("modal?"=TRUE, "eingabe"="Bitte Passwort eingeben") -> ("ok"=w665:bool, "String 3"=w668:string)  [unwired: 8 out]
                  n188 = Increment(x=w667) -> (x+1=w666:i32)
                }
                frame 1 {
                  n189 = case shown="True" w675 {
                    tunnel: [0 w685] -> w676
                    tunnel: w674 -> [w677 w682]
                    tunnel: [w677 w683] -> w673
                    tunnel: w672 -> [_ w680]
                    tunnel: w671 -> [_ w679]
                    frame False {
                    }
                    frame True {
                      n190 = Equal?(x=w682, y="456") -> (x = y?=w684:bool)
                      n191 = case shown="True" w684 {
                        tunnel: [0 1] -> w685
                        tunnel: ["" w688] -> w683
                        tunnel: w682 -> [_ w688]
                        tunnel: w680 -> [_ _]
                        tunnel: w679 -> [_ _]
                        frame False {
                        }
                        frame True {
                          n192 = stacked-sequence {
                            frame #0 {
                              n193 = call "Write Single.vi"("Output_Action"=enum8{"Off", "On"}."On", "Module"=T5."Extension 1", "Single_Output"=T4."Output 3 (O3)", "Output_PWM"=T3."Power 8") -> ()  [unwired: 2 in, 10 out]
                              n194 = call "Write Single.vi"("Output_Action"=enum8{"Off", "On"}."Off", "Module"=T5."Extension 1", "Single_Output"=T4."Output 7 (O7)", "Output_PWM"=T3."Power 8") -> ()  [unwired: 2 in, 10 out]
                            }
                            frame #1 {
                              n195 = call "Verzögerung5"() -> ()  [unwired: 11 in, 1 out]
                            }
                            frame #2 {
                              w698 = FALSE
                              n196 = local write "gesperrt?"(w698) -> ()
                              n197 = local write "Sperren"(w698) -> ()
                            }
                          }
                        }
                      }
                    }
                  }
                }
              }
            }
          }
          n198 = call "Read Single Digital.vi"("Device ID"=w545, "Module"=w544, "Digital_Input"=T6."Input 4 (I4)") -> ("Value"=w541:bool, "error out"=w542:errorcluster)  [unwired: 1 in, 10 out]
          n199 = case shown="True" "schließen" {
            tunnel: [FALSE w635] -> w550
            tunnel: "error in (no error)" -> [_ w634]
            frame False {
            }
            frame True {
              n200 = stacked-sequence {
                tunnel: [_ _ TRUE] -> w635
                tunnel: w634 -> [_ w637 w638]
                tunnel: [_ w636 _] -> w633
                frame #0 {
                  n201 = call "Verzögerung3"() -> ()  [unwired: 2 in, 10 out]
                }
                frame #1 {
                  n202 = call-poly "Close Comm.vi"("error in"=w637) -> ("error out"=w636:errorcluster)  [unwired: 1 in, 13 out]
                }
                frame #2 {
                  n203 = local write "Ende"(TRUE) -> ()
                  n204 = local read "export?"() -> (w641:bool)
                  n205 = case shown="True" w641 {
                    selector: w641 -> [w643 _]
                    tunnel: w638 -> [_ w644]
                    frame False {
                      n206 = Not(x=w643) -> (.not. x?=w642:bool)
                      n207 = Stop(stop? (T)=w642) -> ()
                    }
                    frame True {
                      n208 = control-ref of="dieses VI"() -> (w645:refnum<vi>)
                      n209 = invoke class="\"" method="FP.Schließen"(reference=w645, error in=w644) -> ()  [unwired: 1 in, 3 out]
                    }
                  }
                }
              }
              n210 = local write "error out senke"(w633) -> ()
            }
          }
          n211 = case shown="True" "farbe" {
            tunnel: w545 -> [_ w599]
            tunnel: "error in (no error)" -> [_ w600]
            frame False {
            }
            frame True {
              n212 = flat-sequence {
                tunnel: w600 -> [w604]
                tunnel: w599 -> [w603]
                frame #0 {
                  n213 = local write "gesperrt?"(TRUE ("gesperrt?")) -> ()
                }
                frame #1 {
                  n214 = local read "export?"() -> (w602:bool)
                  n215 = call "Farbanpassung.vi"("error in (no error)"=w604, "modal?"=w602, "Device ID"=w603) -> ("Farbwerte"=→"Farbwerte":T1)  [unwired: 8 out]
                }
                frame #2 {
                  n216 = call "Write Single.vi"("Output_Action"=enum8{"Off", "On"}."On", "Module"=T5."Extension 1", "Single_Output"=T4."Output 3 (O3)", "Output_PWM"=T3."Power 8") -> ()  [unwired: 2 in, 10 out]
                }
                frame #3 {
                  n217 = call "Verzögerung9"() -> ()  [unwired: 2 in, 10 out]
                }
                frame #4 {
                  n218 = local write "gesperrt?"(FALSE ("gesperrt?")) -> ()
                }
              }
            }
          }
          n219 = And(x=w575, y="pneutest") -> (x .and. y?=w576:bool)
          n220 = call "Read Single Digital.vi"("Device ID"=w545, "Module"=w544, "Digital_Input"=T6."Input 5 (I5)", "error in"=w542) -> ("Value"=w540:bool, "error out"=w538:errorcluster)  [unwired: 10 out]
          n221 = call "Read Multi Digital.vi"("Device ID"=w545, "Module"=w571, "Digital Input"=w573) -> ("Value"=w572:bool[], "error out"=w558:errorcluster)  [unwired: 1 in, 10 out]
          n222 = local write "error out senke"(w538) -> ()
          n223 = Unbundle By Name(w558) -> ("status"=w557:bool, "code"=w556:i32)
          n224 = case shown="True" w576 {
            tunnel: w545 -> [_ w630]
            tunnel: "error in (no error)" -> [_ w629]
            frame False {
            }
            frame True {
              n225 = call "Pneumatiktest.vi"("error in (no error)"=w629, "Device ID"=w630) -> ()  [unwired: 10 out]
            }
          }
          n226 = And(x=w541, y=w540) -> (x .and. y?=w539:bool)
          n227 = Array To Cluster(array=w572) -> (cluster=w570:T12)
          n228 = case shown="True" w539 {
            selector: w539 -> [_ w586]
            frame False {
            }
            frame True {
              n229 = local write "gesperrt?"(w586) -> ()
              n230 = local write "Sperren"(w586) -> ()
            }
          }
          n231 = Equal?(x=w556, y=-536866138) -> (x = y?=w554:bool)
          n232 = Unbundle(w570) -> ("Value[0]"=w569:bool, "Value[1]"=w568:bool, "Value[2]"=w567:bool, "Value[3]"=w566:bool, "Value[4]"=w565:bool)  [unwired: 4 out]
          n233 = case shown="True" w557 {
            tunnel: w554 -> [_ w592]
            tunnel: [FALSE w591] -> w551
            frame False {
            }
            frame True {
              n234 = case shown="True" w592 {
                selector: w592 -> [_ w594]
                tunnel: [FALSE w598] -> w591
                frame False {
                }
                frame True {
                  n235 = call "Meldung an Benutzer3"("Enable"=w594) -> ("error out"=w595:errorcluster, "Schließen"=w596:bool)  [unwired: 2 in, 7 out]
                  n236 = local write "schließen"(w596) -> ()
                  n237 = local write "endgültigeschließung"(w596) -> ()
                  n238 = call "Verzögerung10"("error in (no error)"=w595) -> ()  [unwired: 1 in, 10 out]
                  n239 = Not(x=w596) -> (.not. x?=w598:bool)
                  n240 = Not(x=w596) -> (.not. x?=w597:bool)
                  n241 = local write "Ende"(w597) -> ()
                  n242 = global write "globale Variable 1.vi" "ende?"(w597) -> ()
                  n243 = call-poly "Close Comm.vi"() -> ()  [unwired: 2 in, 14 out]
                }
              }
            }
          }
          n244 = Compound Arithmetic op=OR("Stopp", w569, w568, w567, w566, w565) -> (w564:bool)
          n245 = property on="Lampe Notaus" class="Bool. (strikt)"("Visible"=w564) -> ()  [unwired: 2 in, 2 out]
          n246 = case shown="True" w564 {
            selector: w564 -> [_ w611]
            frame False {
            }
            frame True {
              n247 = local write "Stopp"(w611) -> ()
              "stop2" <- w611
            }
          }
          n248 = case shown="True" w564 {
            selector: w564 -> [_ w702]
            tunnel: w545 -> [_ w701]
            tunnel: "error in (no error)" -> [_ w707]
            tunnel: "Stopp" -> [_ w704]
            tunnel: [FALSE TRUE] -> w562
            frame False {
              n249 = local write "Lampe Notaus"(FALSE) -> ()
            }
            frame True {
              n250 = call "all of.vi"("Device ID"=w701) -> ()  [unwired: 11 out]
              n251 = global write "globale Variable 1.vi" "not-aus?"(w702) -> ()
              n252 = stacked-sequence {
                tunnel: w707 -> [_ w732]
                tunnel: w704 -> [w708 _]
                frame #0 {
                  n253 = while {
                    stop <- w709 stop-if-true
                    n254 = stacked-sequence {
                      frame #0 {
                        n255 = call "Verzögerung"() -> ()  [unwired: 2 in, 10 out]
                        n256 = local write "Lampe Notaus"(TRUE) -> ()
                      }
                      frame #1 {
                        n257 = call "Verzögerung2"() -> ()  [unwired: 2 in, 10 out]
                        "Lampe Notaus" <- FALSE
                      }
                    }
                    n258 = local read "stop2"() -> (w709:bool)
                  }
                  n259 = while {
                    tunnel: w708 -> [_]
                    stop <- w717 stop-if-true
                    n260 = local read "Stopp"() -> (w722:bool)
                    n261 = Wait Until Next ms Multiple(millisecond multiple=50) -> ()  [unwired: 1 out]
                    n262 = global write "globale Variable 1.vi" "not-aus?"(w722) -> ()
                    n263 = case shown="False" w722 {
                      tunnel: [0 1] -> w721
                      frame False {
                      }
                      frame True {
                      }
                    }
                    n264 = Not(x=w722) -> (.not. x?=w717:bool)
                    n265 = local read "Device ID Out"() -> (w725:T2)
                    n266 = local write "stop2"(w717) -> ()
                    n267 = Current VI's Menubar() -> (w720:refnum<k9>)
                    n268 = Set Menu Item Info(4:T9 {"Include Shift Key?"=FALSE, "Include Ctrl Key?"=TRUE, "Shortcut Key"="Q"} ("Tastenkombination"), 7:"EXIT" ("x"), 9:w717, 10:"Beenden" ("Objektname"), 11:w720) -> (0:w718:errorcluster, 3:w719:refnum<k9>)  [unwired: 1 in, 1 out]
                    n269 = property on="Licht" class="Bool. (strikt)"("Disabled"=w721) -> ()  [unwired: 2 in, 2 out]
                    n270 = property on="Interfacetest" class="Bool."("Disabled"=w721) -> ()  [unwired: 2 in, 2 out]
                    n271 = property on="protokoll" class="Bool."("Disabled"=w721) -> ()  [unwired: 2 in, 2 out]
                    n272 = property on="pneutest" class="Bool."("Disabled"=w721) -> ()  [unwired: 2 in, 2 out]
                    n273 = property on="farbe" class="Bool."("Disabled"=w721) -> ()  [unwired: 2 in, 2 out]
                    n274 = call "Write Single.vi"("Device ID"=w725, "Output_Action"=enum8{"Off", "On"}."On", "Module"=T5."Extension 1", "Single_Output"=T4."Output 4 (O4)", "Output_PWM"=T3."Power 8") -> ("error out"=w726:errorcluster)  [unwired: 1 in, 9 out]
                    n275 = local write "error in (no error)"(w726) -> ()
                    n276 = Set Menu Item Info(7:"SPERREN" ("x"), 8:w718, 9:w717, 10:"Sperren" ("Objektname"), 11:w719) -> ()  [unwired: 4 out]
                  }
                }
                frame #1 {
                  n277 = call "Write Single.vi"("Output_Action"=enum8{"Off", "On"}."Off", "Module"=T5."Extension 1", "Single_Output"=T4."Output 4 (O4)", "Output_PWM"=T3."Power 8", "error in"=w732) -> ()  [unwired: 1 in, 10 out]
                }
              }
              n278 = Increment(x="Not-Aus betätigt") -> (x+1=w705:dbl)
              n279 = local write "Not-Aus betätigt"(w705) -> ()
            }
          }
          n280 = case shown="False" w551 {
            tunnel: w553 -> [w588 _]
            tunnel: [w588 0] -> w552
            frame False {
            }
            frame True {
            }
          }
          n281 = local read "Ende"() -> (w547:bool)
          n282 = Or(x=w547, y=w550) -> (x .or. y?=w548:bool)
          n283 = global write "globale Variable 1.vi" "not-aus?"(w562) -> ()
          n284 = case shown="True" w548 {
            tunnel: w548 -> [_ w587]
            frame False {
            }
            frame True {
              n285 = global write "globale Variable 1.vi" "ende?"(w587) -> ()
            }
          }
        }
        n286 = while {
          shift-right: [w386] -> _
          shift-left: 0 -> [w387]
          stop <- w389 stop-if-true
          n287 = Wait Until Next ms Multiple(millisecond multiple=50) -> ()  [unwired: 1 out]
          n288 = local read "Device ID Out"() -> (w385:T2)
          n289 = case shown="1" w387 {
            selector: w387 -> [w393 _]
            tunnel: [w392 0] -> w386
            tunnel: w385 -> [w391 w406]
            frame 0, Default {
              n290 = local read "gesperrt?"() -> (w390:bool)
              n291 = case shown="False" w390 {
                tunnel: w393 -> [w400 w404]
                tunnel: [w399 w404] -> w392
                tunnel: w391 -> [w396 _]
                frame False {
                  n292 = call "Read Single Digital.vi"("Device ID"=w396, "Module"=T5."Extension 1", "Digital_Input"=T6."Input 8 (I8)") -> ("Value"=w394:bool, "error out"=w395:errorcluster)  [unwired: 1 in, 10 out]
                  n293 = case shown="False" w394 {
                    tunnel: w400 -> [w401 w403]
                    tunnel: [w401 w402] -> w399
                    frame False {
                    }
                    frame True {
                      n294 = Increment(x=w403) -> (x+1=w402:i32)
                    }
                  }
                  n295 = local write "error out senke"(w395) -> ()
                }
                frame True {
                }
              }
            }
            frame 1 {
              n296 = call "baustein_einzug.vi"("Device ID"=w406) -> ("error out"=w405:errorcluster)  [unwired: 1 in, 9 out]
              n297 = local write "error out senke"(w405) -> ()
            }
          }
          n298 = local read "Ende"() -> (w389:bool)
        }
        n299 = local read "error in (no error)"() -> (w381:errorcluster)
        n300 = local read "Device ID Out"() -> (w380:T2)
        n301 = call "Lichtansteuerung.vi"("error in (no error)"=w381, "Device ID"=w380) -> ("error out"=w382:errorcluster)  [unwired: 1 in, 8 out]
        n302 = local write "error in (no error)"(w382) -> ()
      }
    }
  }
  n303 = local write "bearbeitung gestartedt"(w4) -> ()
  n304 = local write "Not-Aus betätigt"(w4) -> ()
  n305 = local write "fehlbearbeitungen"(w4) -> ()
  n306 = local write "Ende"(w5) -> ()
  n307 = local write "endgültigeschließung"(w5) -> ()
  n308 = Not(x=w3) -> (.not. x?=w2:bool)
  n309 = property on="Stopp 2" class="Bool."("Visible"=w2) -> ()  [unwired: 2 in, 2 out]
  "export?" <- w3
  "version" <- "1.5.2.1 beta"
